vi "timestamp test.vi"() -> ()   [LabVIEW 2009]
panel:
  in  "IP address":string
  out "name":string
  out "port":u16
  out "(received)":string
  in  "stop":bool
  out "date/time (sent)":string
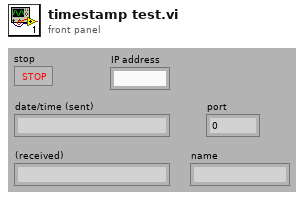
[diagram p1: front panel]
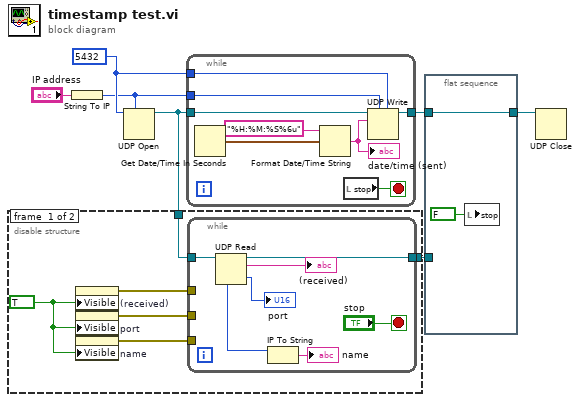
[diagram p0: block diagram]
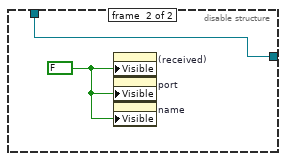
[diagram p2: hidden frame]
diagram:
  w7 = u16 5432 ("port")
  n1 = String To IP(1:"IP address") -> (0:w1:u32)
  n2 = UDP Open(7:w1, 11:w7) -> (port=w6:refnum<k16>)  [unwired: 3 in, 2 out]
  n3 = disable-structure shown="Enabled" {
    disable-tunnel: w6 -> [w13 w21]
    disable-tunnel: [w12 w21] -> w5
    frame #0 {
      w11 = TRUE ("Visible")
      n4 = property on="(received)" class="Str"("Visible"=w11) -> (error out=w8:errorcluster)  [unwired: 2 in, 1 out]
      n5 = property on="port" class="DigNum (strict)"("Visible"=w11) -> (error out=w9:errorcluster)  [unwired: 2 in, 1 out]
      n6 = property on="name" class="Str"("Visible"=w11) -> (error out=w10:errorcluster)  [unwired: 2 in, 1 out]
      n7 = while {
        tunnel: w13 -> [w19]
        tunnel: [w17] -> w12
        tunnel: w10 -> [_]
        tunnel: w9 -> [_]
        tunnel: w8 -> [_]
        stop <- "stop" stop-if-true
        n8 = UDP Read(connection ID=w19) -> (data out=→"(received)":string, 3:w17:refnum<k16>, 4:→"port":u16, 6:w16:u32)  [unwired: 3 in, 1 out]
        n9 = IP To String(2:w16) -> (0:→"name":string)  [unwired: 1 in]
      }
    }
    frame #1 {
      w22 = FALSE ("Visible")
      n10 = property on="(received)" class="Str"("Visible"=w22) -> ()  [unwired: 2 in, 2 out]
      n11 = property on="port" class="DigNum (strict)"("Visible"=w22) -> ()  [unwired: 2 in, 2 out]
      n12 = property on="name" class="Str"("Visible"=w22) -> ()  [unwired: 2 in, 2 out]
    }
  }
  n13 = while {
    tunnel: w6 -> [w30]
    tunnel: [w29] -> w4
    tunnel: w1 -> [w28]
    tunnel: w7 -> [w27]
    stop <- w23 stop-if-true
    n14 = Get Date/Time In Seconds() -> (seconds since 1Jan1904=w26:timestamp)
    n15 = Format Date/Time String(time format string (%c)="%H:%M:%S%6u", seconds (now)=w26) -> (date/time string=w24:string)  [unwired: 1 in]
    "date/time (sent)" <- w24
    n16 = local read "stop"() -> (w23:bool)
    n17 = UDP Write(address=w28, port or service name=w27, connection ID=w30, data in=w24) -> (3:w29:refnum<k16>)  [unwired: 2 in, 1 out]
  }
  n18 = flat-sequence {
    tunnel: w5 -> [_]
    tunnel: w4 -> [w32]
    tunnel: [w32] -> w3
    frame #0 {
      n19 = local write "stop"(FALSE ("stop")) -> ()
    }
  }
  n20 = UDP Close(connection ID=w3) -> ()  [unwired: 1 in, 2 out]
